vi "Clear Report.vi"(8 "error in (no error)":errorcluster, 11 "OnTheFlyReport in":refnum<class "OnTheFlyReport.lvclass">) -> (0 "error out":errorcluster, 3 "OnTheFlyReport out":refnum<class "OnTheFlyReport.lvclass">)   [LabVIEW 2015, in "OnTheFlyReport.lvclass"]
doc: "For on-the-fly reporting, this VI does not do anything."
uses:
  OnTheFlyReport.lvclass
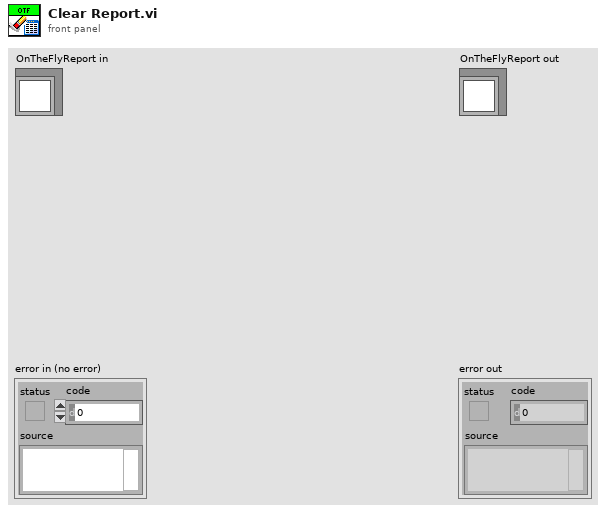
[diagram p1: front panel]
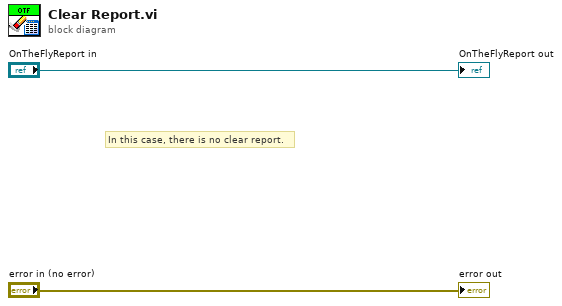
[diagram p0: block diagram]
diagram:
  # "In this case, there is no clear report."
  "error out" <- "error in (no error)"
  "OnTheFlyReport out" <- "OnTheFlyReport in"
